vi "Move to Next Obstacle.vi"(5 "Positon Array":T1[][](array[typedef]), 7 "Map":string[][](array[string]), 10 "Direction":T2, 11 "Start Postion":T1) -> (1 "Positions Covered Out":T1[](array[typedef]), 2 "OFF Grid Out":bool, 3 "End Position Out":T1)   [LabVIEW 2024]
uses:
  Cluster_Position.ctl
  ENUM_Direction.ctl
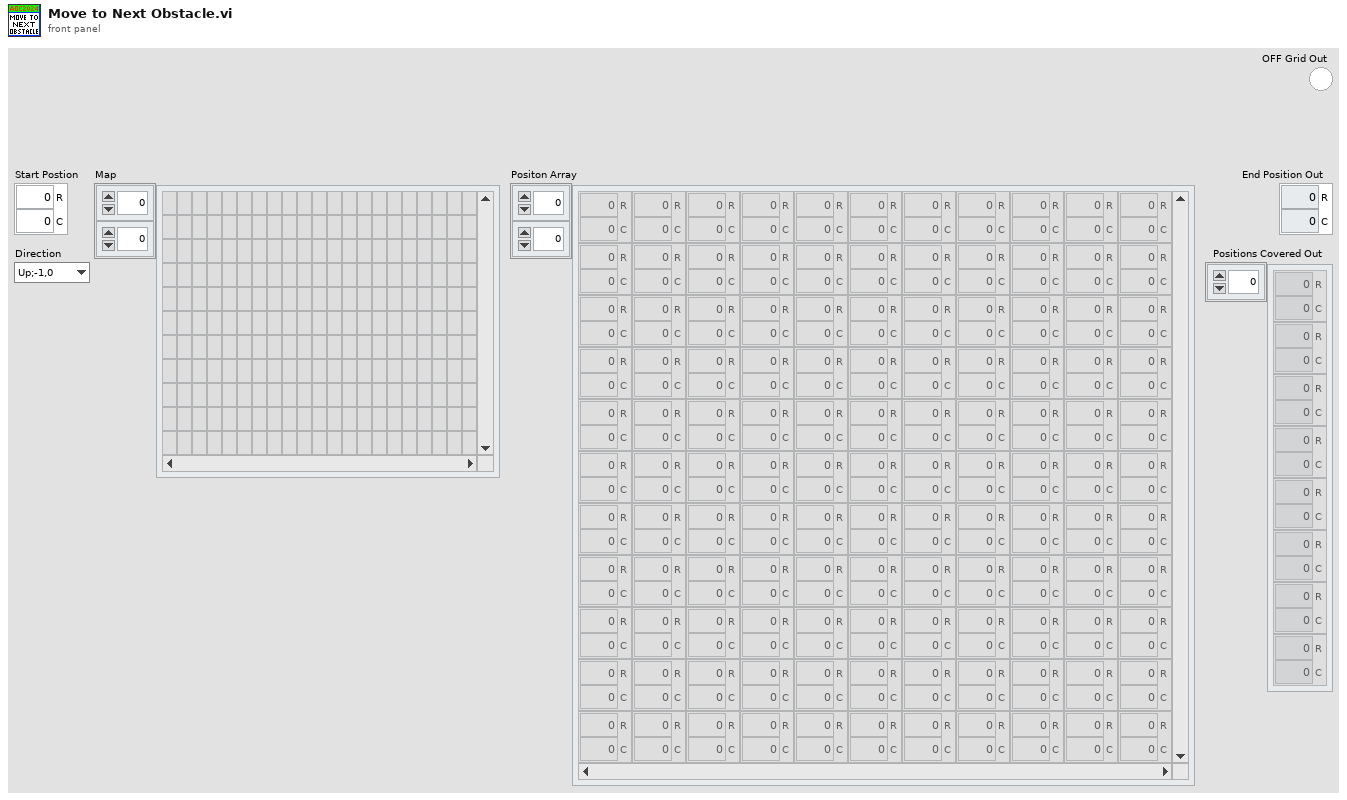
[diagram p1: front panel]
types:
  T1 = typedef "Cluster_Position.ctl" = cluster{"R":i32, "C":i32}
  T2 = typedef "ENUM_Direction.ctl" = enum16{"Up;-1,0", "Right;0,1", "Down;1,0", "Left;0,-1"}
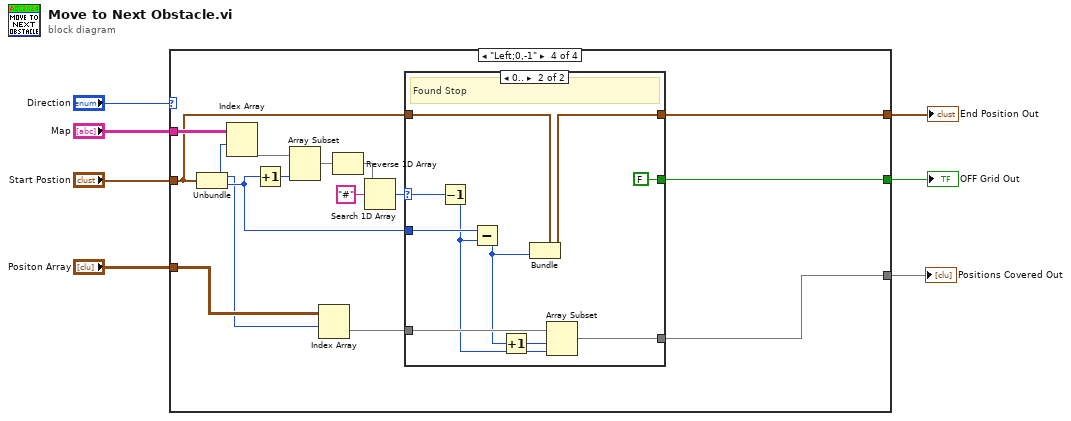
[diagram p0: block diagram]
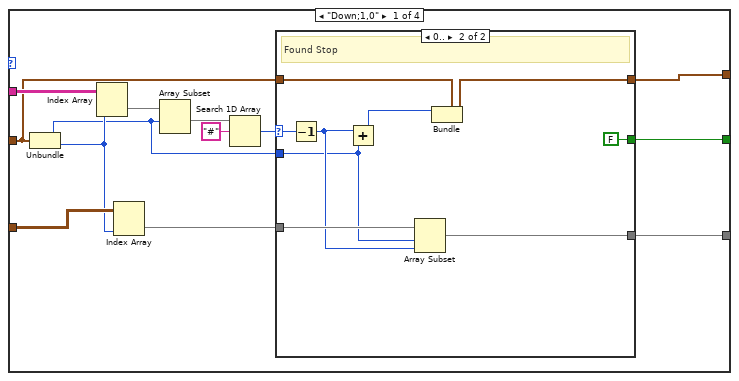
[diagram p2: hidden frame]
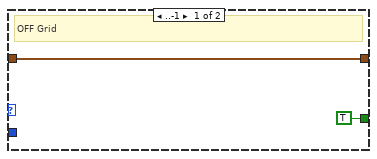
[diagram p3: hidden frame]
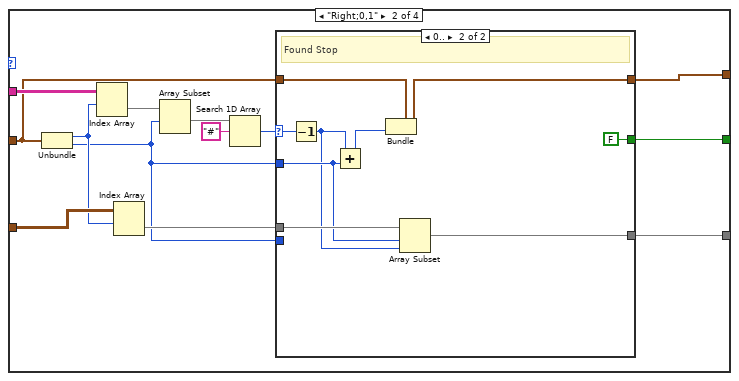
[diagram p4: hidden frame]
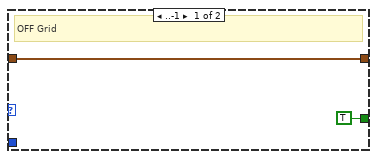
[diagram p5: hidden frame]
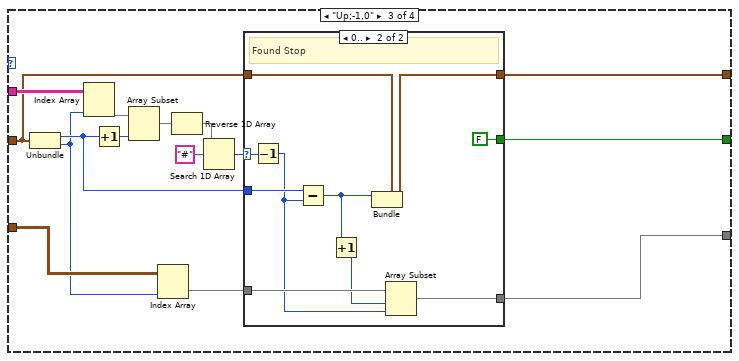
[diagram p6: hidden frame]
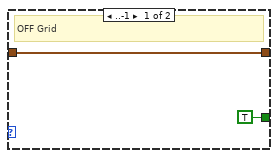
[diagram p7: hidden frame]
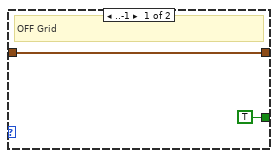
[diagram p8: hidden frame]
diagram:
  n1 = case shown="\"Left;0,-1\"" "Direction" {
    tunnel: "Map" -> [w20 w44 w70 w97]
    tunnel: "Start Postion" -> [w15 w34 w67 w85]
    tunnel: [w16 w40 w68 w95] -> w6
    tunnel: [w14 w39 w66 w94] -> w7
    tunnel: "Positon Array" -> [w13 w38 w60 w88]
    tunnel: [w8 w35 w57 w86] -> w4
    frame "Down;1,0" {
      n2 = Unbundle(w15) -> ("R"=w10:i32, "C"=w12:i32)
      n3 = Index Array(array=w20, index (col)=w12) -> (element=w19:string[])  [unwired: 1 in]
      n4 = Index Array(array=w13, index (col)=w12) -> (element=w11:T1[])  [unwired: 1 in]
      n5 = Array Subset(array=w19, index=w10) -> (w18:string[])  [unwired: 1 in]
      n6 = Search 1D Array(1D array=w18, element="#") -> (index of element=w9:i32)  [unwired: 1 in]
      n7 = case shown="0.." w9 {
        selector: w9 -> [_ w28]
        tunnel: [TRUE FALSE] -> w16
        tunnel: w15 -> [w21 w31]
        tunnel: [w21 w30] -> w14
        tunnel: w11 -> [_ w29]
        tunnel: w10 -> [_ w23]
        tunnel: [_ w27] -> w8
        frame ..-1 {
          # "OFF Grid"
        }
        frame 0.. {
          # "Found Stop"
          n8 = Decrement(x=w28) -> (x-1=w25:i32)
          n9 = Add(x=w25, y=w23) -> (x+y=w24:i32)
          n10 = Array Subset(array=w29, index=w23, length=w25) -> (w27:T1[])
          n11 = Bundle(cluster=w31, "R"=w24) -> (w30:T1)  [unwired: 1 in]
        }
      }
    }
    frame "Right;0,1" {
      n12 = Unbundle(w34) -> ("R"=w33:i32, "C"=w32:i32)
      n13 = Index Array(array=w44, index (row)=w33) -> (element=w43:string[])  [unwired: 1 in]
      n14 = Index Array(array=w38, index (row)=w33) -> (element=w37:T1[])  [unwired: 1 in]
      n15 = Array Subset(array=w43, index=w32) -> (w42:string[])  [unwired: 1 in]
      n16 = Search 1D Array(1D array=w42, element="#") -> (index of element=w36:i32)  [unwired: 1 in]
      n17 = case shown="0.." w36 {
        selector: w36 -> [_ w48]
        tunnel: [TRUE FALSE] -> w40
        tunnel: w34 -> [w45 w55]
        tunnel: [w45 w54] -> w39
        tunnel: w37 -> [_ w53]
        tunnel: w32 -> [_ _]
        tunnel: [_ w52] -> w35
        tunnel: w32 -> [_ w49]
        frame ..-1 {
          # "OFF Grid"
        }
        frame 0.. {
          # "Found Stop"
          n18 = Decrement(x=w48) -> (x-1=w47:i32)
          n19 = Add(x=w47, y=w49) -> (x+y=w50:i32)
          n20 = Bundle(cluster=w55, "C"=w50) -> (w54:T1)  [unwired: 1 in]
          n21 = Array Subset(array=w53, index=w49, length=w47) -> (w52:T1[])
        }
      }
    }
    frame "Up;-1,0" {
      n22 = Unbundle(w67) -> ("R"=w58:i32, "C"=w56:i32)
      n23 = Index Array(array=w70, index (col)=w56) -> (element=w65:string[])  [unwired: 1 in]
      n24 = Increment(x=w58) -> (x+1=w64:i32)
      n25 = Array Subset(array=w65, length=w64) -> (w63:string[])  [unwired: 1 in]
      n26 = Index Array(array=w60, index (col)=w56) -> (element=w59:T1[])  [unwired: 1 in]
      n27 = Reverse 1D Array(array=w63) -> (reversed array=w62:string[])
      n28 = Search 1D Array(1D array=w62, element="#") -> (index of element=w61:i32)  [unwired: 1 in]
      n29 = case shown="0.." w61 {
        selector: w61 -> [_ w77]
        tunnel: [TRUE FALSE] -> w68
        tunnel: w67 -> [w72 w82]
        tunnel: [w72 w81] -> w66
        tunnel: w59 -> [_ w80]
        tunnel: w58 -> [_ w76]
        tunnel: [_ w79] -> w57
        frame ..-1 {
          # "OFF Grid"
        }
        frame 0.. {
          # "Found Stop"
          n30 = Decrement(x=w77) -> (x-1=w75:i32)
          n31 = Subtract(x=w76, y=w75) -> (x-y=w74:i32)
          n32 = Increment(x=w74) -> (x+1=w73:i32)
          n33 = Bundle(cluster=w82, "R"=w74) -> (w81:T1)  [unwired: 1 in]
          n34 = Array Subset(array=w80, index=w73, length=w75) -> (w79:T1[])
        }
      }
    }
    frame "Left;0,-1" {
      n35 = Unbundle(w85) -> ("R"=w83:i32, "C"=w84:i32)
      n36 = Index Array(array=w97, index (row)=w83) -> (element=w93:string[])  [unwired: 1 in]
      n37 = Increment(x=w84) -> (x+1=w92:i32)
      n38 = Array Subset(array=w93, length=w92) -> (w91:string[])  [unwired: 1 in]
      n39 = Index Array(array=w88, index (row)=w83) -> (element=w87:T1[])  [unwired: 1 in]
      n40 = Reverse 1D Array(array=w91) -> (reversed array=w90:string[])
      n41 = Search 1D Array(1D array=w90, element="#") -> (index of element=w89:i32)  [unwired: 1 in]
      n42 = case shown="0.." w89 {
        selector: w89 -> [_ w107]
        tunnel: [TRUE FALSE] -> w95
        tunnel: w85 -> [w99 w109]
        tunnel: [w99 w108] -> w94
        tunnel: w87 -> [_ w106]
        tunnel: w84 -> [_ w105]
        tunnel: [_ w103] -> w86
        frame ..-1 {
          # "OFF Grid"
        }
        frame 0.. {
          # "Found Stop"
          n43 = Decrement(x=w107) -> (x-1=w104:i32)
          n44 = Subtract(x=w105, y=w104) -> (x-y=w101:i32)
          n45 = Increment(x=w101) -> (x+1=w100:i32)
          n46 = Bundle(cluster=w109, "C"=w101) -> (w108:T1)  [unwired: 1 in]
          n47 = Array Subset(array=w106, index=w100, length=w104) -> (w103:T1[])
        }
      }
    }
  }
  "End Position Out" <- w7
  "OFF Grid Out" <- w6
  "Positions Covered Out" <- w4
